vi "_TEST Fields.vi"(4 "error in (no error)":errorcluster) -> (0 "error out":errorcluster)   [LabVIEW 2011]
uses:
  Sequences/Sequence Record.ctl
  Field Record.ctl
  Field DataTypes.ctl
  Field NextItem.ctl
panel:
  out "Field Array Out":T1[](array[typedef])
  out "Field Array Out":T1[](array[typedef])
  out "Field Record":T1={"ixField"=0, "iSequenceOrder"=0, "sxFieldId"="", "sxSequenceId"="", "sDisplayName"="", "sValue"="", "sUnits"="", "nDataType"=enum."timestamp", "nNextItem"=enum."Reset", "fSystem"=FALSE, "fSystemValue"=FALSE, "fRequired"=FALSE, "fSetAtTest"=FALSE, "fTestField"=FALSE, "fDeleted"=FALSE, "fIndexed"=FALSE, "fFreeList"=FALSE}
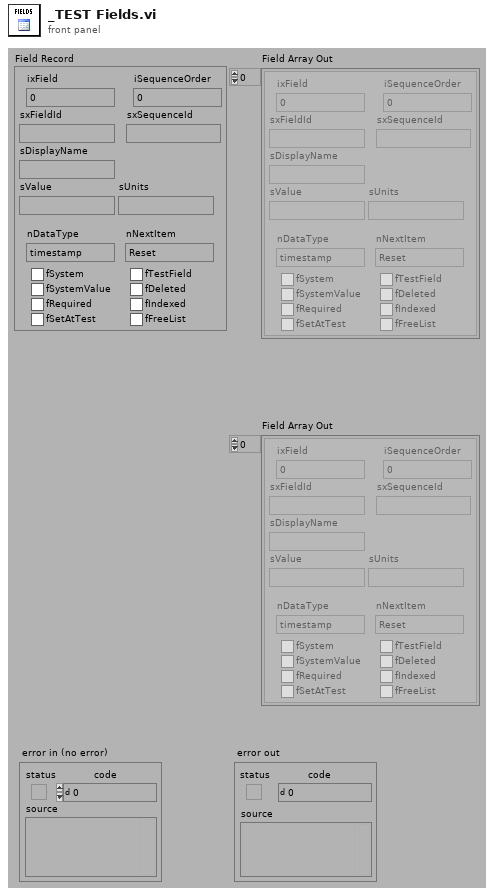
[diagram p1: front panel]
types:
  T1 = typedef "Field Record.ctl" = cluster{"ixField":i32, "iSequenceOrder":i32, "sxFieldId":string, "sxSequenceId":string, "sDisplayName":string, "sValue":string, "sUnits":string, "nDataType":T2, "nNextItem":T3, "fSystem":bool, "fSystemValue":bool, "fRequired":bool, "fSetAtTest":bool, "fTestField":bool, "fDeleted":bool, "fIndexed":bool, "fFreeList":bool}
  T2 = typedef "Field DataTypes.ctl" = enum32{"text", "numeric", "list", "timestamp", "boolean"}
  T3 = typedef "Field NextItem.ctl" = enum32{"Reset", "Retain", "Auto-Increment"}
  T4 = typedef "Sequence Record.ctl" = cluster{"ixSequence":i32, "sxSequenceId":string, "sDescription":string, "sCreator":string, "tCreationDate":timestamp, "sModifier":string, "tModifiedDate":timestamp, "fApproved":bool, "fSpartanSetsSN":bool, "fOverwriteData":bool, "fStopOnFail":bool, "fDisableQuickMode":bool, "fPartialExecution":bool, "fAutoNextItem":bool, "fDoNotPrintOnFail":bool}
  T5 = typedef "Connection Refnum.ctl" = cluster{"Environment Handle":i32, "Connection Handle":i32}
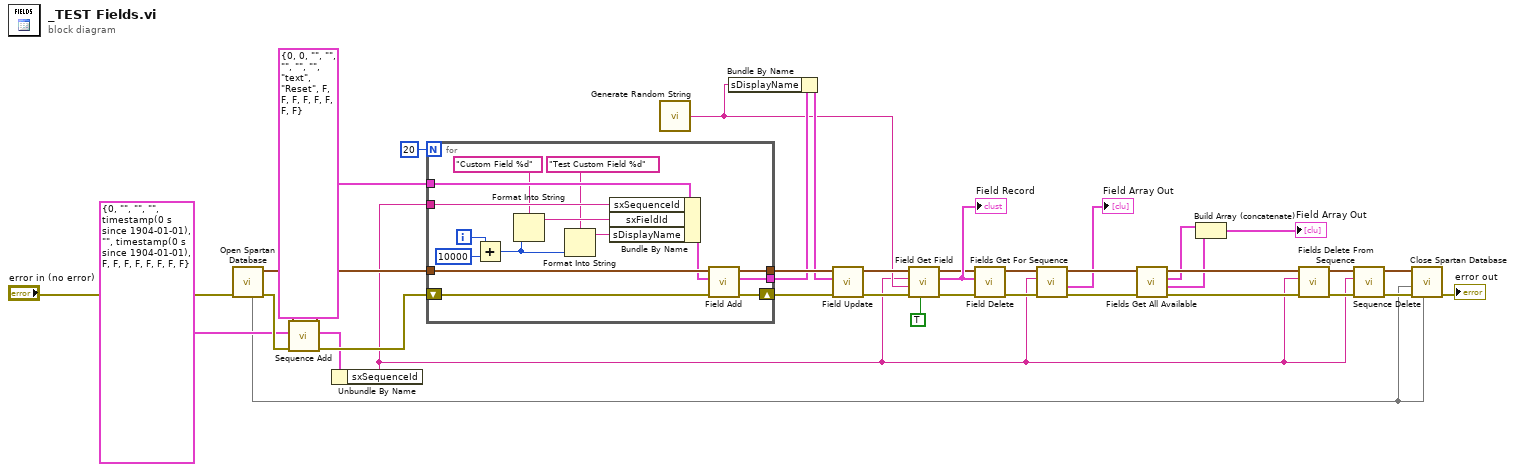
[diagram p0: block diagram]
diagram:
  n1 = call "Open Spartan Database.vi"("error in (no error)"="error in (no error)") -> ("error out"=w33:errorcluster, "Connection Refnum"=w31:T5, 4:w12)  [unwired: 1 in, 7 out]
  n2 = call "Sequence Add.vi"("error in (no error)"=w33, "Sequence Record"=T4 {"ixSequence"=0, "sxSequenceId"="", "sDescription"="", "sCreator"="", "tCreationDate"=timestamp(0 s since 1904-01-01), "sModifier"="", "tModifiedDate"=timestamp(0 s since 1904-01-01), "fApproved"=FALSE, "fSpartanSetsSN"=FALSE, "fOverwriteData"=FALSE, "fStopOnFail"=FALSE, "fDisableQuickMode"=FALSE, "fPartialExecution"=FALSE, "fAutoNextItem"=FALSE, "fDoNotPrintOnFail"=FALSE}, "Connection Refnum"=w31) -> ("error out"=w29:errorcluster, "New Sequence Record"=w28:T4, "Connection Refnum"=w30:T5)  [unwired: 6 out]
  n3 = Unbundle By Name(w28) -> ("sxSequenceId"=w6:string)
  n4 = for {
    N: 20 -> [_]
    tunnel: w30 -> [w52]
    shift-right: [w48] -> w24
    shift-left: w29 -> [w49]
    tunnel: T1 {"ixField"=0, "iSequenceOrder"=0, "sxFieldId"="", "sxSequenceId"="", "sDisplayName"="", "sValue"="", "sUnits"="", "nDataType"=enum."text", "nNextItem"=enum."Reset", "fSystem"=FALSE, "fSystemValue"=FALSE, "fRequired"=FALSE, "fSetAtTest"=FALSE, "fTestField"=FALSE, "fDeleted"=FALSE, "fIndexed"=FALSE, "fFreeList"=FALSE} ("Field Record") -> [w51]
    tunnel: w6 -> [w50]
    tunnel: [w40] -> w25
    tunnel: [w38] -> w23
    i -> [w43]
    n5 = Add(x=w43, y=10000) -> (x+y=w41:i32)
    n6 = Format Into String(format string="Custom Field %d", w41) -> (resulting string=w46:string)  [unwired: 2 in, 1 out]
    n7 = Format Into String(format string="Test Custom Field %d", w41) -> (resulting string=w44:string)  [unwired: 2 in, 1 out]
    n8 = Bundle By Name(cluster=w51, "sxSequenceId"=w50, "sxFieldId"=w46, "sDisplayName"=w44) -> (w39:T1)
    n9 = call "Field Add.vi"("error in (no error)"=w49, "Field Record"=w39, "Connection Refnum"=w52) -> ("error out"=w48:errorcluster, "New Field"=w38:T1, "Connection Refnum"=w40:T5)  [unwired: 1 in, 5 out]
  }
  n10 = call "Generate Random String.vi"() -> ("Output String"=w14:string)  [unwired: 1 in, 4 out]
  n11 = Bundle By Name(cluster=w23, "sDisplayName"=w14) -> (w20:T1)
  n12 = call "Field Update.vi"("error in (no error)"=w24, "Field Record"=w20, "Connection Refnum"=w25) -> ("error out"=w21:errorcluster, "Connection Refnum"=w22:T5)  [unwired: 7 out]
  n13 = call "Field Get Field.vi"("by sDisplayName? (f, by sFieldId)"=TRUE, "error in (no error)"=w21, "sFieldId or sDisplayName (\"\")"=w14, "sxSequenceId (\"\")"=w6, "Connection Refnum"=w22) -> ("error out"=w17:errorcluster, "Field"=w19:T1, "Connection Refnum"=w18:T5)  [unwired: 4 out]
  "Field Record" <- w19
  n14 = call "Field Delete.vi"("error in (no error)"=w17, "Field"=w19, "Connection Refnum"=w18) -> ("error out"=w7:errorcluster, "Connection Refnum"=w9:T5)  [unwired: 7 out]
  n15 = call "Fields Get For Sequence.vi"("error in (no error)"=w7, "sxSequenceId (\"\")"=w6, "Connection Refnum"=w9) -> ("error out"=w5:errorcluster, "Current Sequence Fields"=→"Field Array Out":T1[], "Connection Refnum"=w8:T5)  [unwired: 6 out]
  n16 = call "Fields Get All Available.vi"("error in (no error)"=w5, "Connection Refnum"=w8) -> ("error out"=w11:errorcluster, "Custom Fields"=w2:T1[], "System or ALL Combined Fields"=w3:T1[], "Connection Refnum"=w10:T5)  [unwired: 3 in, 3 out]
  n17 = Build Array (concatenate)(w3, w2) -> (→"Field Array Out":T1[])
  n18 = call "Fields Delete From Sequence.vi"("error in (no error)"=w11, "sxSequenceId (\"\")"=w6, "Connection Refnum"=w10) -> ("error out"=w35:errorcluster, "Connection Refnum"=w37:T5)  [unwired: 7 out]
  n19 = call "Sequence Delete.vi"("error in (no error)"=w35, "Sequence ID"=w6, "Connection Refnum"=w37) -> ("error out"=w34:errorcluster, "Connection Refnum"=w36:T5)  [unwired: 7 out]
  n20 = call "Close Spartan Database.vi"("Force Close? (f)"=w12, "error in (no error)"=w34, 9:w12, "Connection Refnum"=w36) -> ("error out"=→"error out":errorcluster)  [unwired: 1 in, 6 out]
